vi "Update Buffer Words.vi"(6 "data word to write":u16[](array[numeric]), 8 "error in":errorcluster, 9 "buffer type":T1(ring)=enum."BC Message Buffer", 10 "buffer id":u16=1, 11 "module handle":u32) -> (0 "error out":errorcluster, 3 "module handle out":u32)   [LabVIEW 2020, in "AIM MIL-STD-1553 Hardware API.lvlib"]
uses:
  AIM MIL-STD-1553 Hardware API.lvlib
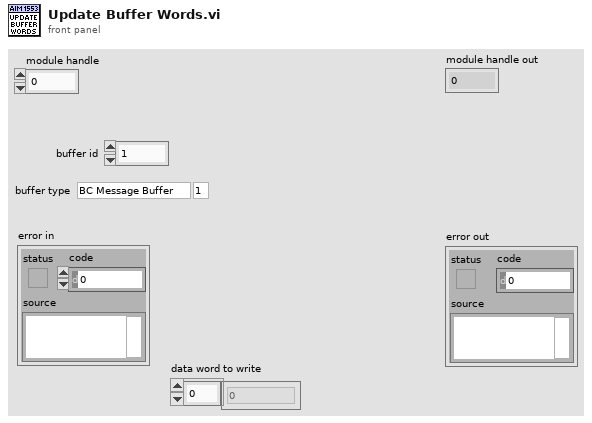
[diagram p1: front panel]
types:
  T1 = enum16{"unknown", "BC Message Buffer", "RT Message Buffer"}
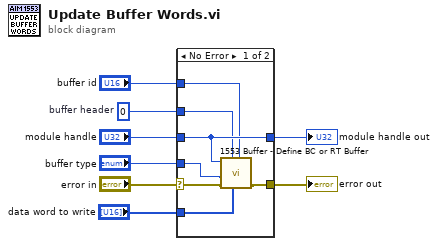
[diagram p0: block diagram]
diagram:
  w1 = u16 0  # buffer header
  n1 = case shown="No Error" "error in" {
    selector: "error in" -> [w15 w17]
    tunnel: [w14 w17] -> w8
    tunnel: "module handle" -> [w11 w16]
    tunnel: "buffer type" -> [w12 _]
    tunnel: "buffer id" -> [w10 _]
    tunnel: "data word to write" -> [w13 _]
    tunnel: [w11 w16] -> w2
    tunnel: w1 -> [w9 _]
    frame No Error {
      n2 = call <instrlib>:"1553 Buffer - Define BC or RT Buffer.vi"("Buffer ID (1)"=w10, "Data Array (32 words, all zero)"=w13, "Buffer Header ID (1)"=w9, "Error In (none)"=w15, "Buffer Type (BC)"=w12, "Module Handle"=w11) -> ("Error Out"=w14:errorcluster)  [unwired: 2 in, 3 out]
    }
    frame Error {
    }
  }
  "error out" <- w8
  "module handle out" <- w2
